vi "Loop.vi"(11 "Template Event in":refnum<class "Template Event.lvclass">) -> (3 "Template Event out":refnum<class "Template Event.lvclass">)   [LabVIEW 2021, in "Template Event.lvlib" / "Template Event.lvclass"]
uses:
  Template Event.lvclass
  C:/Program Files/National Instruments/LabVIEW 2021/vi.lib/Nathan Davis/jettl/jettl/jettl/jettl.lvclass
  Template Event.lvclass/Template Event.ctl
  <vilib>/Nathan Davis/jettl/jettl/Event/Event.lvclass
  <vilib>/Nathan Davis/jettl/jettl/Msg Strategy/Msg Strategy.lvclass
  C:/Program Files/National Instruments/LabVIEW 2021/vi.lib/Nathan Davis/jettl/jettl Msg Merge Error/jettl Msg Merge Error/jettl Msg Merge Error.lvclass
  C:/Program Files/National Instruments/LabVIEW 2021/vi.lib/Nathan Davis/jettl/jettl/Event/Event.lvclass
  C:/Program Files/National Instruments/LabVIEW 2021/vi.lib/Nathan Davis/jettl/jettl Msg Override Error/jettl Msg Override Error/jettl Msg Override Error.lvclass
  C:/Program Files/National Instruments/LabVIEW 2021/vi.lib/Nathan Davis/jettl/jettl Msg Setup/jettl Msg Setup/jettl Msg Setup.lvclass
  C:/Program Files/National Instruments/LabVIEW 2021/vi.lib/Nathan Davis/jettl/jettl Msg Teardown/jettl Msg Teardown/jettl Msg Teardown.lvclass
  C:/Program Files/National Instruments/LabVIEW 2021/vi.lib/Nathan Davis/jettl/jettl/jettl Msg Last Ack Creator Queue/jettl Msg Last Ack Creator Queue/jettl Msg Last Ack Creator Queue.lvclass
  C:/git/jettl/jettl Tools/_Template/Templates/Template Event/Template Event/Template Event.lvclass
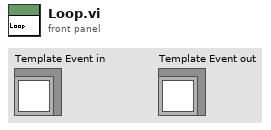
[diagram p1: front panel]
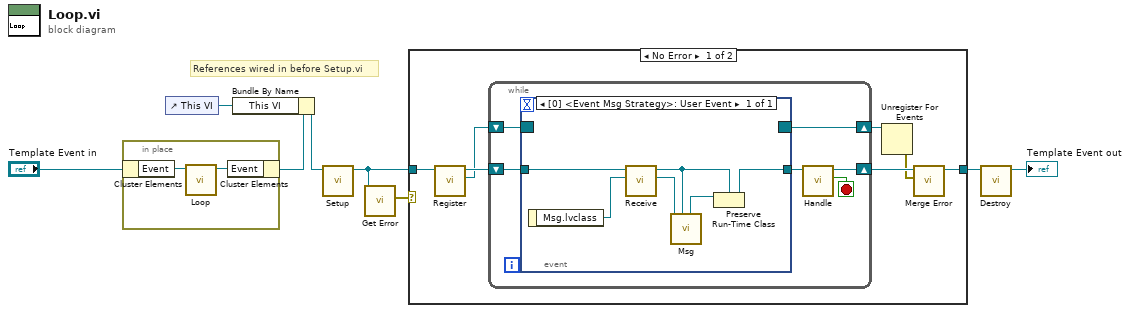
[diagram p0: block diagram]
diagram:
  # "References wired in before Setup.vi"
  n1 = in-place {
    n2 = in-place-cluster #1("Template Event in") -> ("Event"=w10:refnum<class "Event.lvclass">)
    n3 = call-dynamic "Loop.vi"("Event in"=w10) -> ("Event out"=w9:refnum<class "Event.lvclass">)  [unwired: 10 in]
    n4 = in-place-cluster #1("Event"=w9) -> (w7:refnum<class "Template Event.lvclass">)
  }
  n5 = control-ref of="This VI"() -> (w6:refnum<vi>)
  n6 = Bundle By Name(cluster=w7, "This VI"=w6) -> (w5:refnum<class "Template Event.lvclass">)
  n7 = call-dynamic "Setup.vi"("Template Event in"=w5) -> ("Template Event out"=w3:refnum<class "Template Event.lvclass">)  [unwired: 10 in]
  n8 = call-dynamic "Get Error.vi"("Template Event in"=w3) -> ("Error"=w4:errorcluster)  [unwired: 10 in]
  n9 = case shown="No Error" w4 {
    tunnel: w3 -> [w17 w30]
    tunnel: [w12 w30] -> w2
    frame No Error {
      n10 = call-dynamic "Register.vi"("Template Event in"=w17) -> ("Registration"=w14:refnum<event-registration>, "Template Event out"=w15:refnum<class "Template Event.lvclass">)  [unwired: 9 in]
      n11 = while {
        shift-right: [w22] -> w16
        shift-left: w14 -> [w23]
        shift-right: [w19] -> w13
        shift-left: w15 -> [w21]
        stop <- w18 stop-if-true
        n12 = event shown="[0] <Event Msg Strategy>: User Event" {
          selector: w23 -> [_]
          dyn-events: [_] -> w22
          timeout: _ -> [_]
          tunnel: w21 -> [w27]
          tunnel: [w29] -> w20
          event User Event {
            n13 = event-data() -> ("Msg.lvclass"=w24:refnum<class "Msg Strategy.lvclass">)  [unwired: 1 in]
            n14 = call-dynamic "Receive.vi"("Msg Strategy in"=w24, "Template Event in"=w27) -> ("Msg Strategy out"=w25:refnum<class "Msg Strategy.lvclass">, "Template Event out"=w26:refnum<class "Template Event.lvclass">)  [unwired: 8 in]
            n15 = call-dynamic "Msg.vi"("jettl in"=w26, "Msg Strategy in"=w25) -> ("jettl out"=w28:refnum<class "jettl.lvclass">)  [unwired: 9 in]
            n16 = Preserve Run-Time Class(object in=w28, 2:w26) -> (object out=w29:refnum<class "Template Event.lvclass">)  [unwired: 1 in, 1 out]
          }
        }
        n17 = call-dynamic "Handle.vi"("Template Event in"=w20) -> ("Destroy?"=w18:bool, "Template Event out"=w19:refnum<class "Template Event.lvclass">)  [unwired: 9 in]
      }
      n18 = Unregister For Events(event registration refnum=w16) -> (error out=w11:errorcluster)  [unwired: 1 in]
      n19 = call-dynamic "Merge Error.vi"("Error"=w11, "Template Event in"=w13) -> ("Template Event out"=w12:refnum<class "Template Event.lvclass">)  [unwired: 9 in]
    }
    frame Error {
    }
  }
  n20 = call-dynamic "Destroy.vi"("Template Event in"=w2) -> ("Template Event out"=→"Template Event out":refnum<class "Template Event.lvclass">)  [unwired: 10 in]
